vi "Cache SSH Fingerprint.vi"(8 "error in (no error)":errorcluster, 11 "HPS17000 IP Address":string) -> (0 "error out":errorcluster, 3 "result":bool)   [LabVIEW 2023, in "HPS-17000-PowerModule.lvlib" / "HPS-17000-PowerModule.lvclass"]
uses:
  HPS-17000-PowerModule.lvclass
  <vilib>/net/SSH/Client/PuTTY/PuTTY Client.lvclass
  C:/Program Files/National Instruments/LabVIEW 2023/vi.lib/net/SSH/Client/Generic/Generic Client.lvclass
  <vilib>/net/SSH/Client/Generic/Generic Client.lvclass/Generic Client.ctl
  <vilib>/net/SSH/Client/Generic/Write trust on first use.vi
  <vilib>/net/SSH/NI_SSH.lvlib
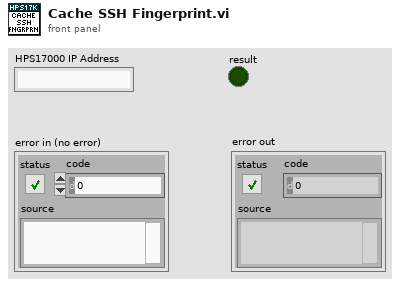
[diagram p1: front panel]
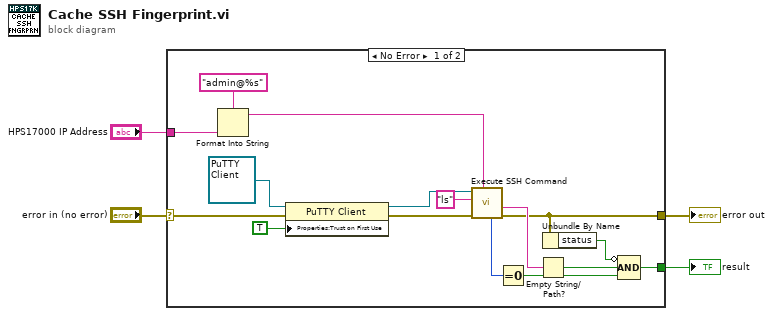
[diagram p0: block diagram]
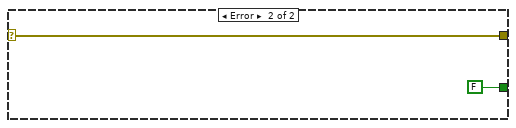
[diagram p2: hidden frame]
diagram:
  n1 = case shown="No Error" "error in (no error)" {
    selector: "error in (no error)" -> [w6 w22]
    tunnel: "HPS17000 IP Address" -> [w15 _]
    tunnel: [w9 w22] -> w3
    tunnel: [w7 FALSE] -> w2
    frame No Error {
      n2 = Format Into String(format string="admin@%s", w15) -> (resulting string=w20:string)  [unwired: 2 in, 1 out]
      n3 = property class="PuTTY Client"(reference=refnum<class "PuTTY Client.lvclass"> refnum ("NI_SSH.lvlib:PuTTY Client"), error in=w6, "Properties:Trust on First Use"=TRUE ("Trust on First Use")) -> (reference out=w17:refnum<class "PuTTY Client.lvclass">, error out=w16:errorcluster)
      n4 = call <vilib>:"Execute SSH Command.vi"("user@host"=w20, "error in (no error)"=w16, "command line"="ls", "session in"=w17) -> ("error out"=w9:errorcluster, "standard error"=w13:string, "return code"=w12:i32)  [unwired: 3 in, 2 out]
      n5 = Equal To 0?(x=w12) -> (x = 0?=w10:bool)
      n6 = Empty String/Path?(string/path=w13) -> (empty?=w11:bool)
      n7 = Unbundle By Name(w9) -> ("status"=w8:bool)
      n8 = Compound Arithmetic op=AND(invert w8, w11, w10) -> (w7:bool)
    }
    frame Error {
    }
  }
  "error out" <- w3
  "result" <- w2
